vi "7SPOTMEAS_loopnov_2.vi"() -> ()   [LabVIEW 2020]
panel:
  in  "Channel":u16(ring) items=["1", "2"]
  in  "stop":bool
  out "Waveform Chart":dbl(graph)
  in  "VISA resource name":refnum<visa-resource-name>
  out "Measurement Result":dbl
  in  "Measurement Mode (0:Voltage)":enum16{"Voltage", "Current", "Resistance"}(ring)
  # "CURRENT IN mA\nVOLTAGE IN V\nRESISTANCE IN Ohms"
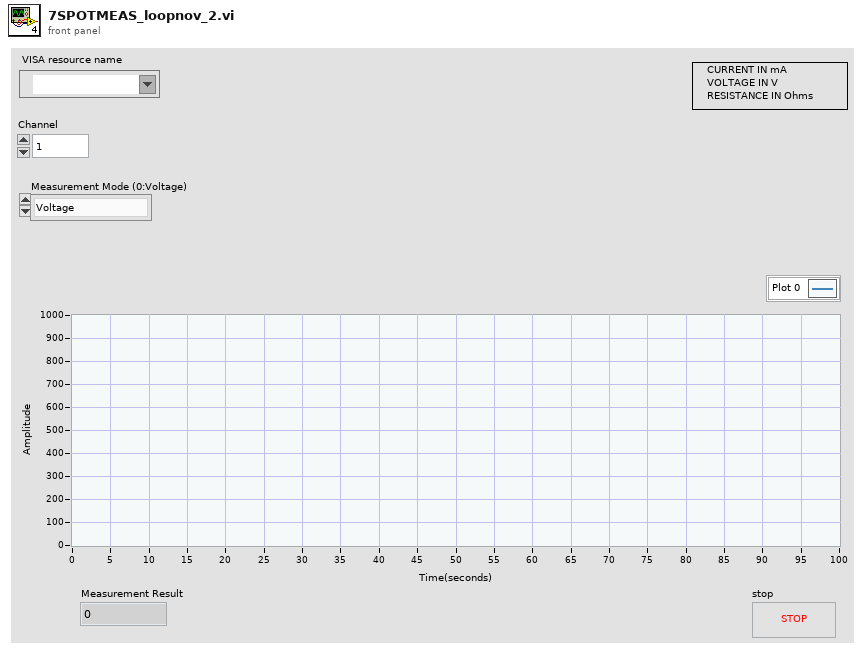
[diagram p1: front panel]
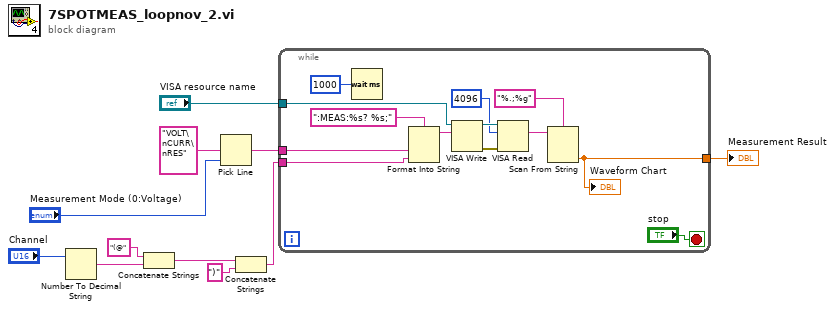
[diagram p0: block diagram]
diagram:
  n1 = Number To Decimal String(number="Channel") -> (decimal integer string=w6:string)  [unwired: 1 in]
  n2 = Concatenate Strings("(@", w6) -> (w5:string)
  n3 = Pick Line(multi-line string="VOLT\nCURR\nRES", line index="Measurement Mode (0:Voltage)") -> (output string=w11:string)  [unwired: 1 in]
  n4 = Concatenate Strings(w5, ")") -> (w2:string)
  n5 = while {
    tunnel: w11 -> [w22]
    tunnel: "VISA resource name" -> [w16]
    tunnel: w2 -> [w15]
    tunnel: [w12] -> w3
    stop <- "stop" stop-if-true
    n6 = Wait (ms)(milliseconds to wait=u32 1000) -> ()  [unwired: 1 out]
    n7 = Format Into String(format string=":MEAS:%s? %s;", w22, w15) -> (resulting string=w21:string)  [unwired: 2 in, 1 out]
    n8 = VISA Write(VISA resource name=w16, write buffer=w21) -> (VISA resource name out=w18:refnum<visa-resource-name>, error out=w19:errorcluster)  [unwired: 1 in, 1 out]
    n9 = VISA Read(VISA resource name=w18, byte count=u32 4096, error in (no error)=w19) -> (read buffer=w24:string)  [unwired: 3 out]
    n10 = Scan From String(format string="%.;%g", input string=w24) -> (output 1=w12:dbl)  [unwired: 3 in, 3 out]
    "Waveform Chart" <- w12
  }
  "Measurement Result" <- w3
